vi "15.2.2 MultiGeoMatch.vi"() -> ()   [LabVIEW 2016]
uses:
  <vilib>/vision/Image Controls.llb/IMAQ Image.ctl
  <vilib>/vision/Pattern Matching.llb/IMAQ GM Match Report.ctl
  <vilib>/vision/Pattern Matching.llb/IMAQ GM Multiple Template.ctl
  <vilib>/vision/Pattern Matching.llb/IMAQ Match Range Setting.ctl
  <vilib>/vision/NI_Vision_Development_Module.lvlib
panel:
  out "Bracket Matches":i32
  out "Plate Matches":i32
  out "Hanger Matches":i32
  in  "Bracket Color":u32(colorbox)=16711680
  in  "Plate Color":u32(colorbox)=6618880
  in  "Hanger Color":u32(colorbox)=3381759
  out "Hanger":T1(plugin-control)
  out "Plate":T1(plugin-control)
  out "UUT":T1(plugin-control)
  out "Bracket":T1(plugin-control)
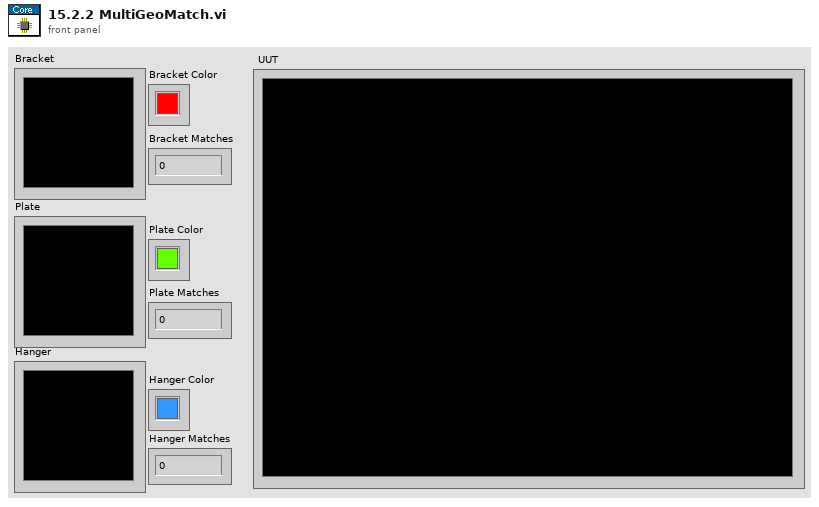
[diagram p1: front panel]
types:
  T1 = typedef "IMAQ Image.ctl" = refnum<image>
  T2 = typedef "IMAQ Match Range Setting.ctl" = cluster{"Match Constraints":u32, "Min":dbl, "Max":dbl}
  T3 = typedef "IMAQ GM Multiple Template.ctl" = refnum<k20>
  T4 = typedef "IMAQ GM Match Report.ctl" = cluster{"Position":cluster{"x":sgl, "y":sgl}, "Angle":sgl, "Scale":sgl, "Score":sgl, "Bounding Box":cluster{"x":sgl, "y":sgl}[], "Contrast Reversed":bool, "Occlusion %":sgl, "Template Target Curve Score":sgl, "Target Template Curve Score":sgl, "Correlation Score":sgl}
  T5 = cluster{"TMPs":T1[], "UUT":T1, "Matches":T4[], "TmpRefs":T3}
  T6 = cluster{"Rotation":bool, "Scale":bool, "Occlusion":bool, "Reserved":bool, "Reserved":bool, "Reserved":bool}
  T7 = cluster{"Match Geometric Pattern Setup Data":string, "Number of Matches":i32, "Minimum Match Score":sgl}
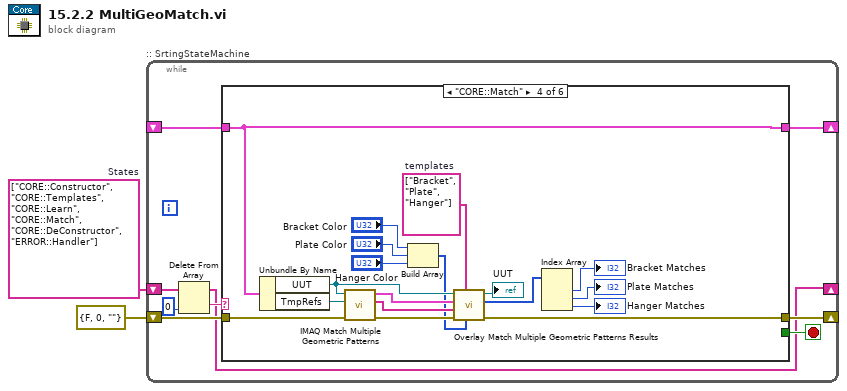
[diagram p0: block diagram]
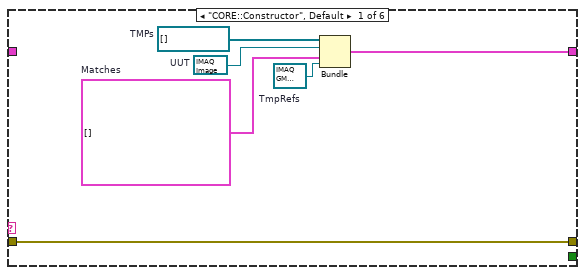
[diagram p2: hidden frame]
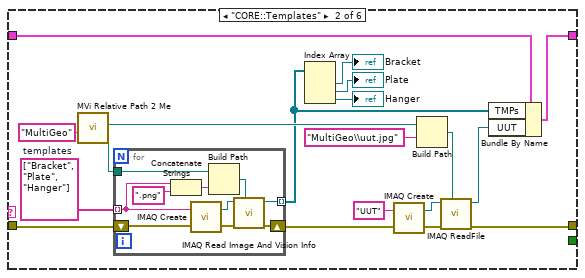
[diagram p3: hidden frame]
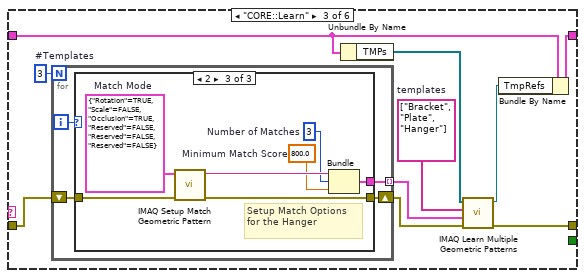
[diagram p4: hidden frame]
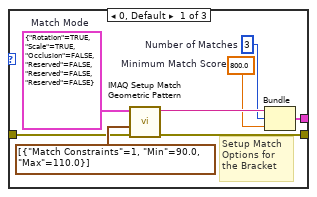
[diagram p5: hidden frame]
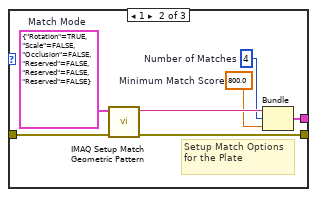
[diagram p6: hidden frame]
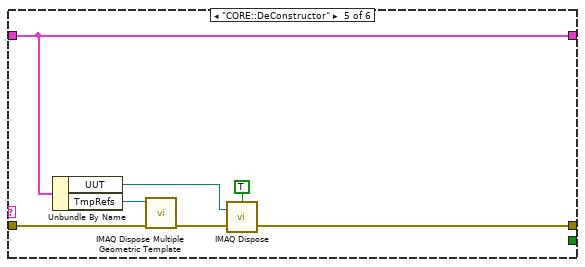
[diagram p7: hidden frame]
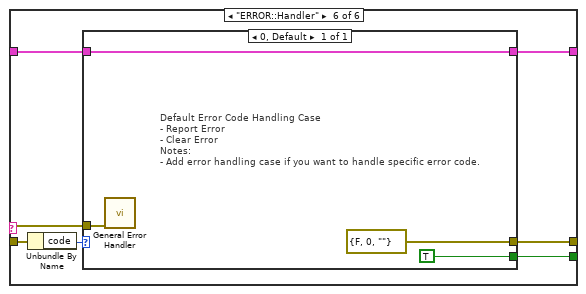
[diagram p8: hidden frame]
diagram:
  w1 = string[] ["CORE::Constructor", "CORE::Templates", "CORE::Learn", "CORE::Match", "CORE::DeConstructor", "ERROR::Handler"]  # States
  n1 = while ":: SrtingStateMachine" {
    shift-right: [w8] -> _
    shift-left: errorcluster {"status"=FALSE, "code"=0, "source"=""} ("ErrI") -> [w6]
    shift-right: [w10] -> _
    shift-left: _ -> [w9]
    shift-right: [w3] -> _
    shift-left: w1 -> [w7]
    stop <- w11 stop-if-true
    n2 = Delete From Array(array=w7, index=0) -> (deleted portion=w5:string, array with subset deleted=w3:string[])  [unwired: 1 in]
    n3 = case shown="\"CORE::Match\"" w5 {
      tunnel: [w16 w25 w50 w97 w106 w110] -> w8
      tunnel: [_ _ _ _ _ w109] -> w11
      tunnel: w6 -> [w16 w34 w53 w100 w104 w108]
      tunnel: [w17 w35 w55 w84 w107 w111] -> w10
      tunnel: w9 -> [_ w36 w56 w84 w107 w112]
      frame "CORE::Constructor", Default {
        w12 = T3 refnum  # TmpRefs
        w13 = T1[] []  # TMPs
        w14 = T4[] []  # Matches
        w15 = T1 refnum  # UUT
        n4 = Bundle("TMPs"=w13, "UUT"=w15, "Matches"=w14, "TmpRefs"=w12) -> (w17:T5)  [unwired: 1 in]
      }
      frame "CORE::Templates" {
        w33 = string[] ["Bracket", "Plate", "Hanger"]  # templates
        n5 = call "MVi Relative Path 2 Me.vi"("Relative Path"="MultiGeo") -> ("Appended Dir"=w31:path, "MyDir"=w21:path)  [unwired: 5 in]
        n6 = for {
          tunnel: w33 -> [w42] mode=indexing
          tunnel: w31 -> [w46]
          tunnel: [w43] -> w18 mode=indexing
          shift-right: [w38] -> w26
          shift-left: w34 -> [w37]
          n7 = Concatenate Strings(w42, ".png" ("string")) -> (w41:string)
          n8 = call "IMAQ Create"("Image Name"=w42, "error in (no error)"=w37) -> ("Src"=w44:T1, "error out"=w39:errorcluster)  [unwired: 3 in]
          n9 = Build Path(base path=w46, name or relative path=w41) -> (appended path=w45:path)
          n10 = call "IMAQ Read Image And Vision Info"("File Path"=w45, "error in (no error)"=w39, "Image"=w44) -> ("error out"=w38:errorcluster, "Image Out"=w43:T1)  [unwired: 6 in, 1 out]
        }
        n11 = Index Array(array=w18) -> (element #1=→"Bracket":T1, element #2=→"Plate":T1, element #3=→"Hanger":T1)  [unwired: 3 in]
        n12 = call "IMAQ Create"("Image Name"="UUT", "error in (no error)"=w26) -> ("Src"=w24:T1, "error out"=w27:errorcluster)  [unwired: 3 in]
        n13 = Build Path(base path=w21, name or relative path="MultiGeo\\uut.jpg" ("Relative Path")) -> (appended path=w20:path)
        n14 = call "IMAQ ReadFile"("File Path"=w20, "error in (no error)"=w27, "Image"=w24) -> ("error out"=w25:errorcluster, "Image Out"=w19:T1)  [unwired: 4 in, 3 out]
        n15 = Bundle By Name(cluster=w36, "TMPs"=w18, "UUT"=w19) -> (w35:T5)
      }
      frame "CORE::Learn" {
        w48 = string[] ["Bracket", "Plate", "Hanger"]  # templates
        w54 = 3  # #Templates
        n16 = for {
          N: w54 -> [_]
          tunnel: [w60] -> w52 mode=indexing
          shift-right: [w58] -> w51
          shift-left: w53 -> [w57]
          i -> [w59]
          n17 = case shown="2" w59 {
            tunnel: [w65 w72 w79] -> w60
            tunnel: [w62 w69 w76] -> w58
            tunnel: w57 -> [w61 w70 w77]
            frame 0, Default {
              w63 = T6 {"Rotation"=TRUE, "Scale"=TRUE, "Occlusion"=FALSE, "Reserved"=FALSE, "Reserved"=FALSE, "Reserved"=FALSE}  # Match Mode
              w66 = sgl 800.0  # Minimum Match Score
              w67 = 3  # Number of Matches
              # "Setup Match Options for the Bracket"
              n18 = call "IMAQ Setup Match Geometric Pattern"("error in (no error)"=w61, "Range Settings"=T2[] [{"Match Constraints"=1, "Min"=90.0, "Max"=110.0}], "Match Mode"=w63) -> ("error out"=w62:errorcluster, "Match Geometric Pattern Setup Data"=w68:string)  [unwired: 7 in]
              n19 = Bundle("Match Geometric Pattern Setup Data"=w68, "Number of Matches"=w67, "Minimum Match Score"=w66) -> (w65:T7)  [unwired: 1 in]
            }
            frame 1 {
              w71 = T6 {"Rotation"=TRUE, "Scale"=FALSE, "Occlusion"=FALSE, "Reserved"=FALSE, "Reserved"=FALSE, "Reserved"=FALSE}  # Match Mode
              w73 = sgl 800.0  # Minimum Match Score
              w74 = 4  # Number of Matches
              # "Setup Match Options for the Plate"
              # "Setup Match Options for the Plate Template"
              n20 = call "IMAQ Setup Match Geometric Pattern"("error in (no error)"=w70, "Match Mode"=w71) -> ("error out"=w69:errorcluster, "Match Geometric Pattern Setup Data"=w75:string)  [unwired: 8 in]
              n21 = Bundle("Match Geometric Pattern Setup Data"=w75, "Number of Matches"=w74, "Minimum Match Score"=w73) -> (w72:T7)  [unwired: 1 in]
            }
            frame 2 {
              w78 = T6 {"Rotation"=TRUE, "Scale"=FALSE, "Occlusion"=TRUE, "Reserved"=FALSE, "Reserved"=FALSE, "Reserved"=FALSE}  # Match Mode
              w80 = sgl 800.0  # Minimum Match Score
              w81 = 3  # Number of Matches
              # "Setup Match Options for the Hanger"
              # "Setup Match Options for the Hanger Template"
              n22 = call "IMAQ Setup Match Geometric Pattern"("error in (no error)"=w77, "Match Mode"=w78) -> ("error out"=w76:errorcluster, "Match Geometric Pattern Setup Data"=w82:string)  [unwired: 8 in]
              n23 = Bundle("Match Geometric Pattern Setup Data"=w82, "Number of Matches"=w81, "Minimum Match Score"=w80) -> (w79:T7)  [unwired: 1 in]
            }
          }
        }
        n24 = Unbundle By Name(w56) -> ("TMPs"=w49:T1[])
        n25 = call "IMAQ Learn Multiple Geometric Patterns"("error in (no error)"=w51, "Default Match Options"=w52, "Template Labels"=w48, "Template Images"=w49) -> ("error out"=w50:errorcluster, "Multiple Template (out)"=w47:T3)  [unwired: 6 in]
        n26 = Bundle By Name(cluster=w56, "TmpRefs"=w47) -> (w55:T5)
      }
      frame "CORE::Match" {
        w83 = string[] ["Bracket", "Plate", "Hanger"]  # templates
        n27 = Unbundle By Name(w84) -> ("UUT"=w94:T1, "TmpRefs"=w99:T3)
        n28 = call "IMAQ Match Multiple Geometric Patterns"("error in (no error)"=w100, "Multiple Template"=w99, "Image"=w94) -> ("error out"=w98:errorcluster, "Matched Labels"=w96:string[], "Matches (pixel)"=w95:T4[])  [unwired: 5 in, 1 out]
        n29 = Build Array("Bracket Color", "Plate Color", "Hanger Color") -> (w90:u32[])
        n30 = call "Overlay Match Multiple Geometric Patterns Results.vi"("Label Colors"=w90, "Learned Labels"=w83, "error in"=w98, "Match Labels"=w96, "Match Results"=w95, "Image"=w94) -> ("error out"=w97:errorcluster, "Number of Matches"=w86:i32[], "Image Out"=→"UUT":T1)  [unwired: 3 in]
        n31 = Index Array(array=w86) -> (element #1=→"Bracket Matches":i32, element #2=→"Plate Matches":i32, element #3=→"Hanger Matches":i32)  [unwired: 3 in]
      }
      frame "CORE::DeConstructor" {
        n32 = Unbundle By Name(w107) -> ("UUT"=w105:T1, "TmpRefs"=w101:T3)
        n33 = call "IMAQ Dispose Multiple Geometric Template"("error in (no error)"=w104, "Multiple Template"=w101) -> ("error out"=w103:errorcluster)  [unwired: 9 in]
        n34 = call "IMAQ Dispose"("All Images? (No)"=TRUE, "Image"=w105, "error in (no error)"=w103) -> ("error out"=w106:errorcluster)  [unwired: 3 in]
      }
      frame "ERROR::Handler" {
        n35 = Unbundle By Name(w108) -> ("code"=w113:i32)
        n36 = case shown="0, Default" w113 {
          tunnel: [w117] -> w111
          tunnel: w112 -> [w117]
          tunnel: [errorcluster {"status"=FALSE, "code"=0, "source"=""} ("error out")] -> w110
          tunnel: [TRUE] -> w109
          tunnel: w108 -> [w115]
          frame 0, Default {
            # "Default Error Code Handling Case\n- Report Error\n- Clear Error \nNotes:\n- Add error handling case if you want to handle specific error code."
            n37 = call <vilib>:"General Error Handler.vi"("error in (no error)"=w115) -> ()  [unwired: 10 in, 5 out]
          }
        }
      }
    }
  }
